vi "Virtual-TimeSimulated_EnergySystem.vi"() -> ()   [LabVIEW 2017]
uses:
  classes/DataCollector.lvclass
  classes/DataHandler.lvclass
  classes/SimulationParameter.lvclass
panel:
  out "Th. Sorage Loading":cluster{"Load":bool, "Unload":bool}
  out "El. Sorage Loading":cluster{"Load":bool, "Unload":bool}
  out "Public Grid":bool
  out "Emergency Cooling":bool
  out "Energy flow After Sorages":T1
  out "El. Sorage [kWh]":dbl(slide) scale=0.0..26.1
  out "Th. Sorage [kWh]":dbl(slide) scale=0.0..200.0
  out "Energy flow Befor Sorages":T1
  out "Day of Year":u32
  out "Total Energy \nof System":T1
  out "Day Time":u32
  in  "Time Interval":u32=1
  in  "stop":bool
  # "Virtual-time Simulated CPS-Energy System: TODO: Change it to a Real-Time System"
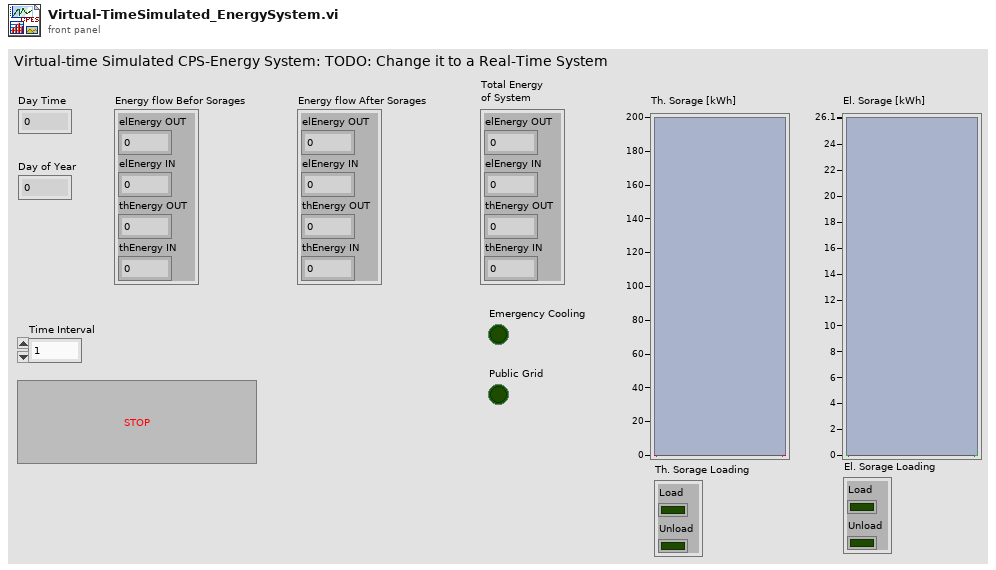
[diagram p1: front panel]
types:
  T1 = cluster{"elEnergy OUT":dbl, "elEnergy IN":dbl, "thEnergy OUT":dbl, "thEnergy IN":dbl}
  T2 = cluster{"DataCollector out":refnum<class "DataCollector.lvclass">, "DataHandler out":refnum<class "DataHandler.lvclass">, "SimulationParameter out":refnum<class "SimulationParameter.lvclass">}
  T3 = cluster{"DataCollector":refnum<class "DataCollector.lvclass">, "DataHandling":refnum<class "DataHandler.lvclass">, "SimulationParameter":refnum<class "SimulationParameter.lvclass">}
  T4 = cluster{"Th. Capacity":dbl, "Th. Charge State":dbl}
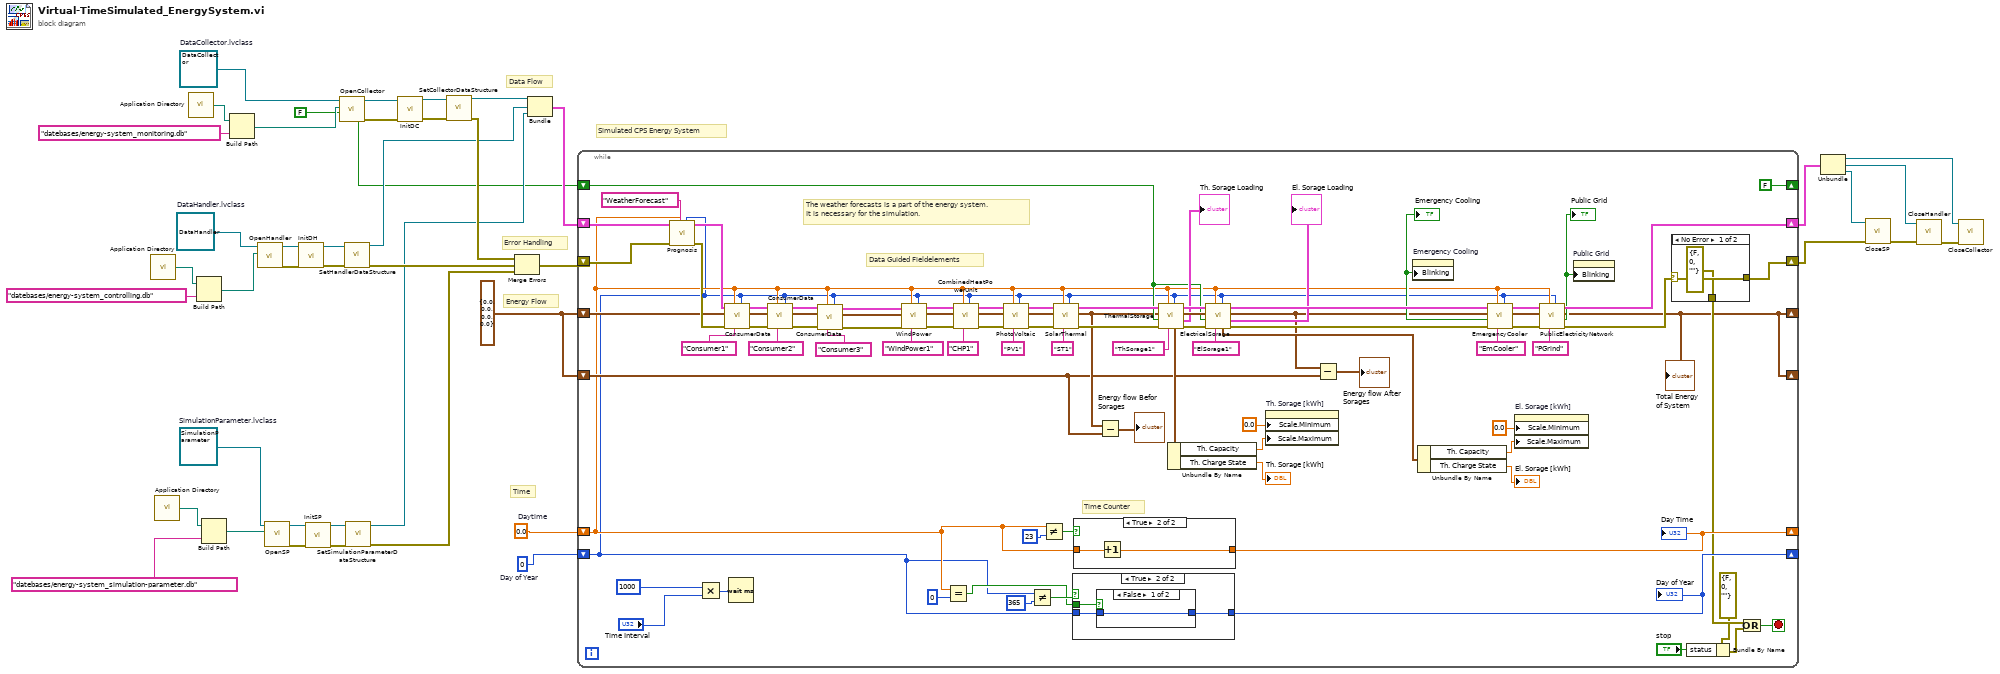
[diagram p0: block diagram]
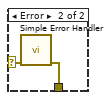
[diagram p2: hidden frame]
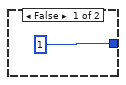
[diagram p3: hidden frame]
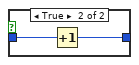
[diagram p4: hidden frame]
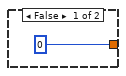
[diagram p5: hidden frame]
diagram:
  w12 = refnum<class "SimulationParameter.lvclass"> refnum  # SimulationParameter.lvclass
  w39 = refnum<class "DataHandler.lvclass"> refnum  # DataHandler.lvclass
  w38 = refnum<class "DataCollector.lvclass"> refnum  # DataCollector.lvclass
  w43 = u32 0  # Day of Year
  w44 = 0.0  # Daytime
  w2 = T1 {"elEnergy OUT"=0.0, "elEnergy IN"=0.0, "thEnergy OUT"=0.0, "thEnergy IN"=0.0} ("Energy flow IN")
  # "Error Handling"
  # "Simulated CPS Energy System"
  # "Data Flow"
  # "Time"
  # "Energy Flow"
  n1 = call <vilib>:"Application Directory.vi"() -> ("Application Directory"=w42:path)
  n2 = call <vilib>:"Application Directory.vi"() -> ("Application Directory"=w16:path)
  n3 = call <vilib>:"Application Directory.vi"() -> ("Application Directory"=w40:path)
  n4 = Build Path(base path=w42, name or relative path="datebases/energy-system_controlling.db" ("Name oder relativer Pfad")) -> (appended path=w41:path)
  n5 = Build Path(base path=w16, name or relative path="datebases/energy-system_simulation-parameter.db" ("Name oder relativer Pfad")) -> (appended path=w11:path)
  n6 = Build Path(base path=w40, name or relative path="datebases/energy-system_monitoring.db" ("Name oder relativer Pfad")) -> (appended path=w4:path)
  n7 = call-dynamic "OpenHandler.vi"("path to db monitoring"=w41, "DataHandling in"=w39) -> ("error out"=w25:errorcluster, "DataHandling out"=w24:refnum<class "DataHandler.lvclass">)  [unwired: 8 in]
  n8 = call-dynamic "OpenSP.vi"("path to db simulation"=w11, "SimulationParameter in"=w12) -> ("error out"=w9:errorcluster, "SimulationParameter out"=w10:refnum<class "SimulationParameter.lvclass">)  [unwired: 8 in]
  n9 = call-dynamic "InitDH.vi"("error in (no error)"=w25, "DataHandler in"=w24) -> ("error out"=w20:errorcluster, "DataHandler out"=w21:refnum<class "DataHandler.lvclass">)  [unwired: 8 in]
  n10 = call-dynamic "InitSP.vi"("error in (no error)"=w9, "SimulationParameter in"=w10) -> ("error out"=w8:errorcluster, "SimulationParameter out"=w7:refnum<class "SimulationParameter.lvclass">)  [unwired: 8 in]
  n11 = call-dynamic "OpenCollector.vi"("Ram?"=FALSE, "path to db monitoring"=w4, "DataCollector in"=w38) -> ("error out"=w26:errorcluster, "Rows = 0?"=w1:bool, "DataCollector out"=w29:refnum<class "DataCollector.lvclass">)  [unwired: 6 in]
  n12 = call-dynamic "SetHandlerDataStructure.vi"("error in (no error)"=w20, "DataHandler in"=w21) -> ("error out"=w18:errorcluster, "DataHandler out"=w19:refnum<class "DataHandler.lvclass">)  [unwired: 8 in]
  n13 = call-dynamic "SetSimulationParameterDataStructure.vi"("error in (no error)"=w8, "SimulationParameter in"=w7) -> ("error out"=w5:errorcluster, "SimulationParameter out"=w6:refnum<class "SimulationParameter.lvclass">)  [unwired: 8 in]
  n14 = call-dynamic "InitDC.vi"("error in (no error)"=w26, "DataCollector in"=w29) -> ("error out"=w27:errorcluster, "DataCollector out"=w28:refnum<class "DataCollector.lvclass">)  [unwired: 8 in]
  n15 = call-dynamic "SetCollectorDataStructure.vi"("error in (no error)"=w27, "DataCollector in"=w28) -> ("error out"=w22:errorcluster, "DataCollector out"=w30:refnum<class "DataCollector.lvclass">)  [unwired: 8 in]
  n16 = Merge Errors(w22, w18, w5) -> (w23:errorcluster)
  n17 = Bundle("DataCollector out"=w30, "DataHandler out"=w19, "SimulationParameter out"=w6) -> (w36:T2)  [unwired: 1 in]
  n18 = while {
    shift-right: [w52] -> _
    shift-left: w2 -> [w82]
    shift-right: [w126] -> _
    shift-left: w44 -> [w46]
    shift-right: [w120] -> _
    shift-left: w43 -> [w45]
    shift-right: [w104] -> w14
    shift-left: w23 -> [w89]
    shift-right: [w109] -> w35
    shift-left: w36 -> [w90]
    shift-right: [FALSE ("Ram?")] -> _
    shift-left: w1 -> [w53]
    shift-right: [w52] -> _
    shift-left: w2 -> [w47]
    stop <- w103 stop-if-true
    # "The weather forecasts is a part of the energy system.\nIt is necessary for the simulation."
    # "Data Guided Fieldelements"
    # "Time Counter"
    n19 = call "Prognosis.vi"("Day of Year"=w45, "Unique Object Identifier"="WeatherForecast", "Day Time"=w46, "Error In"=w89, "DataFlowIN"=w90) -> ("Error Out"=w86:errorcluster, "DataFlowOUT"=w81:T3)  [unwired: 5 in]
    n20 = Multiply(x=u32 1000, y="Time Interval") -> (x*y=w130:u32)
    n21 = call "ConsumerData.vi"("Day of Year"=w45, "Unique Object Identifier"="Consumer1", "Day Time"=w46, "Error In"=w86, "Energy flow IN"=w82, "DataFlowIN"=w81) -> ("Error Out"=w83:errorcluster, "Energy flow OUT"=w84:T1, "DataFlowOUT"=w85:T3)  [unwired: 3 in]
    n22 = Wait (ms)(milliseconds to wait=w130) -> ()  [unwired: 1 out]
    n23 = call "ConsumerData.vi"("Day of Year"=w45, "Unique Object Identifier"="Consumer2", "Day Time"=w46, "Error In"=w83, "Energy flow IN"=w84, "DataFlowIN"=w85) -> ("Error Out"=w74:errorcluster, "Energy flow OUT"=w69:T1, "DataFlowOUT"=w71:T3)  [unwired: 3 in]
    n24 = call "ConsumerData.vi"("Day of Year"=w45, "Unique Object Identifier"="Consumer3", "Day Time"=w46, "Error In"=w74, "Energy flow IN"=w69, "DataFlowIN"=w71) -> ("Error Out"=w73:errorcluster, "Energy flow OUT"=w68:T1, "DataFlowOUT"=w70:T3)  [unwired: 3 in]
    n25 = call "WindPower.vi"("Day of Year"=w45, "Unique Object Identifier"="WindPower1", "Day Time"=w46, "Error In"=w73, "Energy flow IN"=w68, "DataFlowIN"=w70) -> ("Error Out"=w108:errorcluster, "Energy flow OUT"=w107:T1, "DataFlowOUT"=w106:T3)  [unwired: 3 in]
    n26 = Equal?(x=w46, y=u32 0) -> (x = y?=w121:bool)
    n27 = call "CombinedHeatPowerUnit.vi"("Day of Year"=w45, "Unique Object Identifier"="CHP1", "Day Time"=w46, "Error In"=w108, "Energy flow IN"=w107, "DataFlowIN"=w106) -> ("Error Out"=w117:errorcluster, "Energy flow OUT"=w118:T1, "DataFlowOUT"=w119:T3)  [unwired: 3 in]
    n28 = call "PhotoVoltaic.vi"("Day of Year"=w45, "Unique Object Identifier"="PV1", "Day Time"=w46, "Error In"=w117, "Energy flow IN"=w118, "DataFlowIN"=w119) -> ("Error Out"=w116:errorcluster, "Energy flow OUT"=w115:T1, "DataFlowOUT"=w114:T3)  [unwired: 3 in]
    n29 = Not Equal?(x=w45, y=u32 365) -> (x != y?=w124:bool)
    n30 = Not Equal?(x=w46, y=u32 23) -> (x != y?=w123:bool)
    n31 = call "SolarThermal.vi"("Day of Year"=w45, "Unique Object Identifier"="ST1", "Day Time"=w46, "Error In"=w116, "Energy flow IN"=w115, "DataFlowIN"=w114) -> ("Error Out"=w113:errorcluster, "Energy flow OUT"=w49:T1, "DataFlowOUT"=w110:T3)  [unwired: 3 in]
    n32 = case shown="True" w124 {
      tunnel: [u32 1 ("Timer-Wert (ms)") w138] -> w120
      tunnel: w45 -> [_ w137]
      tunnel: w121 -> [_ w136]
      frame False {
      }
      frame True {
        n33 = case shown="False" w136 {
          tunnel: [w139 w141] -> w138
          tunnel: w137 -> [w139 w140]
          frame False {
          }
          frame True {
            n34 = Increment(x=w140) -> (x+1=w141:u32)
          }
        }
      }
    }
    "Day of Year" <- w120
    n35 = case shown="True" w123 {
      tunnel: [u32 0 ("Timer-Wert (ms)") w144] -> w126
      tunnel: w46 -> [_ w143]
      frame False {
      }
      frame True {
        n36 = Increment(x=w143) -> (x+1=w144:dbl)
      }
    }
    "Day Time" <- w126
    n37 = Subtract(x=w49, y=w47) -> (x-y=→"Energy flow Befor Sorages":T1)
    n38 = call "ThermalStorage.vi"("Day of Year"=w45, "Unique Object Identifier"="ThSorage1", "Day Time"=w46, "Error In"=w113, "FirstLoop?"=w53, "Energy flow IN"=w49, "DataFlowIN"=w110) -> ("Error Out"=w59:errorcluster, "Th. Sorage Loading"=→"Th. Sorage Loading":cluster{"Load":bool, "Unload":bool}, "Energy flow OUT"=w112:T1, "DataFlowOUT"=w111:T3, "Sorage Level"=w67:T4)
    n39 = Unbundle By Name(w67) -> ("Th. Capacity"=w65:dbl, "Th. Charge State"=→"Th. Sorage [kWh]":dbl)
    n40 = call "ElectricalSorage.vi"("Day of Year"=w45, "Unique Object Identifier"="ElSorage1", "Day Time"=w46, "Error In"=w59, "FirstLoop?"=w53, "Energy flow IN"=w112, "DataFlowIN"=w111) -> ("Error Out"=w80:errorcluster, "El. Sorage Loading"=→"El. Sorage Loading":cluster{"Load":bool, "Unload":bool}, "Energy flow OUT"=w51:T1, "DataFlowOUT"=w77:T3, "Sorage Level"=w60:T4)
    n41 = property on="Th. Sorage [kWh]" class="Slide (strict)"("Scale.Minimum"=0.0 ("Scale.Range:Minimum"), "Scale.Maximum"=w65) -> ()  [unwired: 2 in, 2 out]
    n42 = Subtract(x=w51, y=w47) -> (x-y=→"Energy flow After Sorages":T1)
    n43 = Unbundle By Name(w60) -> ("Th. Capacity"=w62:dbl, "Th. Charge State"=→"El. Sorage [kWh]":dbl)
    n44 = call "EmergencyCooler.vi"("Day of Year"=w45, "Unique Object Identifier"="EmCooler", "Day Time"=w46, "Error In"=w80, "Energy flow IN"=w51, "DataFlowIN"=w77) -> ("Error Out"=w79:errorcluster, "Emergency cooling"=w58:bool, "Energy flow OUT"=w78:T1, "DataFlowOUT"=w76:T3)  [unwired: 2 in]
    "Emergency Cooling" <- w58
    n45 = property on="Emergency Cooling" class="Bool (strict)"("Blinking"=w58) -> ()  [unwired: 2 in, 2 out]
    n46 = property on="El. Sorage [kWh]" class="Slide (strict)"("Scale.Minimum"=0.0 ("Scale.Range:Minimum"), "Scale.Maximum"=w62) -> ()  [unwired: 2 in, 2 out]
    n47 = call "PublicElectricityNetwork.vi"("Day of Year"=w45, "Unique Object Identifier"="PGrind", "Day Time"=w46, "Error In"=w79, "Energy flow IN"=w78, "DataFlowIN"=w76) -> ("Error Out"=w105:errorcluster, "Feeding into the \npublic grid"=w57:bool, "Energy flow OUT"=w52:T1, "DataFlowOUT"=w109:T3)  [unwired: 2 in]
    "Total Energy \nof System" <- w52
    "Public Grid" <- w57
    n48 = property on="Public Grid" class="Bool (strict)"("Blinking"=w57) -> ()  [unwired: 2 in, 2 out]
    n49 = case shown="No Error" w105 {
      selector: w105 -> [w132 w134]
      tunnel: [w132 _] -> w104
      tunnel: [errorcluster {"status"=FALSE, "code"=0, "source"=""} ("error out") w133] -> w102
      frame No Error {
      }
      frame Error {
        n50 = call <vilib>:"Simple Error Handler.vi"("error in (no error)"=w134) -> ("error out"=w133:errorcluster)  [unwired: 4 in, 4 out]
      }
    }
    n51 = Bundle By Name(cluster=errorcluster {"status"=FALSE, "code"=0, "source"=""} ("error out"), "status"="stop") -> (w99:errorcluster)
    n52 = Or(x=w102, y=w99) -> (x .or. y?=w103:bool)
  }
  n53 = Unbundle(w35) -> ("DataCollector out"=w34:refnum<class "DataCollector.lvclass">, "DataHandler out"=w33:refnum<class "DataHandler.lvclass">, "SimulationParameter out"=w15:refnum<class "SimulationParameter.lvclass">)
  n54 = call-dynamic "CloseSP.vi"("error in (no error)"=w14, "SimulationParameter in"=w15) -> ("error out"=w13:errorcluster)  [unwired: 8 in, 1 out]
  n55 = call-dynamic "CloseHandler.vi"("error in (no error)"=w13, "DataHandling in"=w33) -> ("error out"=w37:errorcluster)  [unwired: 8 in, 1 out]
  n56 = call "CloseCollector.vi"("error in (no error)"=w37, "DataCollector in"=w34) -> ()  [unwired: 8 in, 2 out]
